vi "robot_object_test.vi"() -> ()   [LabVIEW 2009]
uses:
  OGRE/nick/FPGA/behaviors/driveable paths/test variable.vi
panel:
  in  "number 16\" iterations":i32
  in  "y LIDAR position":i16
  in  "x LIDAR position":i16
  out "Y positions":i16[](array[numeric])
  out "x positions":i16[](array[numeric])
  out "XY Graph":cluster{"Y":dbl[], "Y":dbl[]}[](graph)
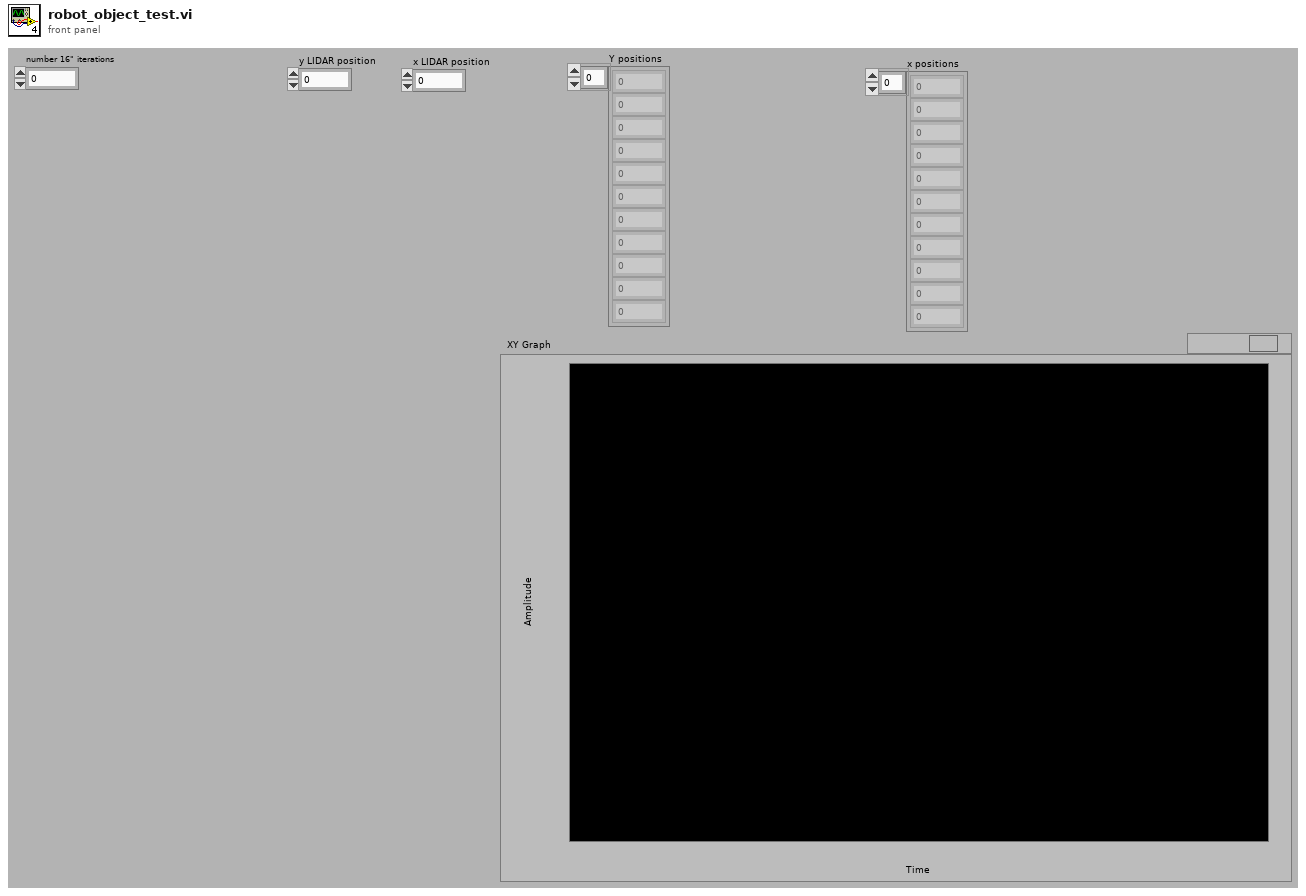
[diagram p1: front panel]
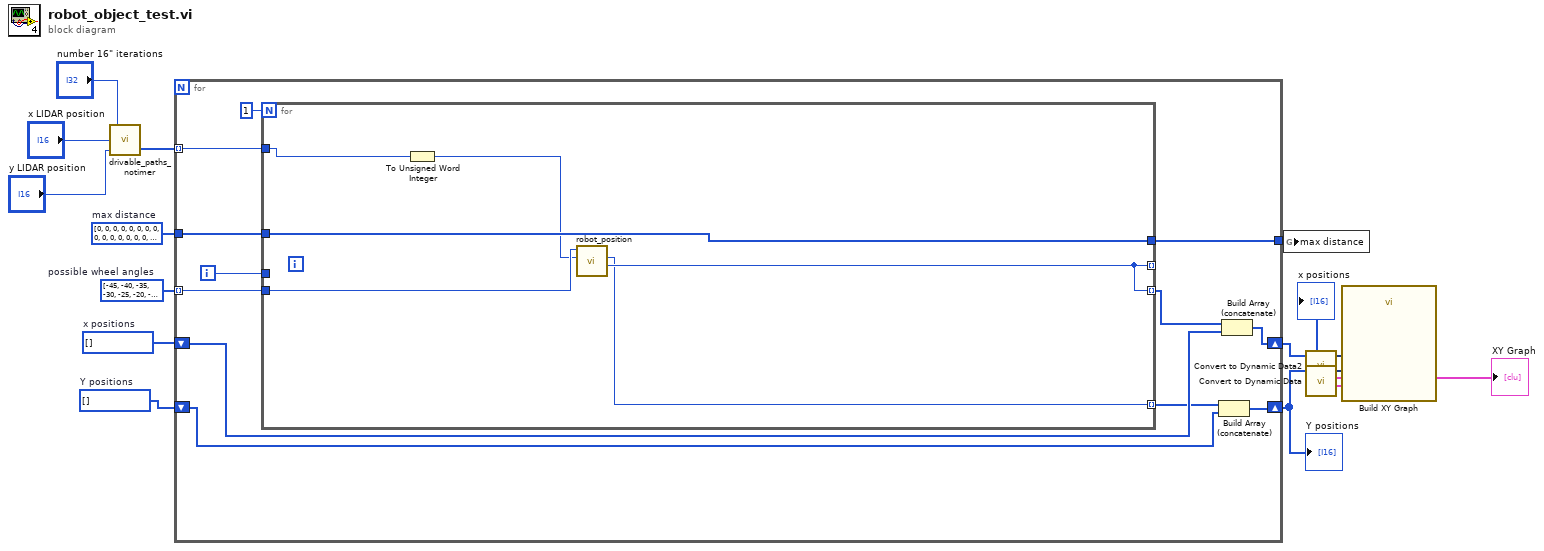
[diagram p0: block diagram]
diagram:
  w9 = i16[] []  # Y positions
  w10 = i16[] []  # x positions
  w12 = i8[] [-45, -40, -35, -30, -25, -20, -15, -10, -5, 0, 5, 10, 15, 20, 25, 30, 35, 40, 45]  # possible wheel angles
  w13 = i16[] [0, 0, 0, 0, 0, 0, 0, 0, 0, 0, 0, 0, 0, 0, 0, 0, 0, 0, 0]  # max distance
  n1 = call "drivable_paths_notimer.vi"("y LIDAR position"="y LIDAR position", "x LIDAR position"="x LIDAR position", "number 16\" iterations"="number 16\" iterations") -> ("max distance"=w4:i16[])  [unwired: 1 in]
  n2 = for {
    tunnel: w13 -> [w26]
    tunnel: w12 -> [w17] mode=indexing
    tunnel: [w24] -> w11
    shift-right: [w21] -> w6
    shift-left: w10 -> [w22]
    shift-right: [w20] -> w8
    shift-left: w9 -> [w18]
    tunnel: w4 -> [w16] mode=indexing
    i -> [w25]
    n3 = for {
      N: 1 -> [_]
      tunnel: w26 -> [w31]
      tunnel: [w31] -> w24
      tunnel: w25 -> [_]
      tunnel: w17 -> [w32]
      tunnel: [w30] -> _ mode=indexing
      tunnel: [w30] -> w23 mode=indexing
      tunnel: [w29] -> w19 mode=indexing
      tunnel: w16 -> [w28]
      n4 = To Unsigned Word Integer(number=w28) -> (unsigned 16bit integer=w27:u16)
      n5 = call "robot_position.vi"("Distance Along Arc"=w27, "Wheel Angle"=w32) -> ("New X Position"=w30:i8, "New Y Position"=w29:i8)  [unwired: 7 in, 1 out]
    }
    n6 = Build Array (concatenate)(w19, w18) -> (w20:i16[])
    n7 = Build Array (concatenate)(w23, w22) -> (w21:i16[])
  }
  "x positions" <- w6
  "Y positions" <- w8
  n8 = global write "test variable.vi" "max distance"(w11) -> ()
  n9 = call "Convert to Dynamic Data2"("Array"=w6) -> ("Dynamic Data Type"=w5:dynamicdata)  [unwired: 3 in]
  n10 = call "Convert to Dynamic Data"("Array"=w8) -> ("Dynamic Data Type"=w7:dynamicdata)  [unwired: 3 in]
  n11 = call "Build XY Graph"("Y Input"=w7, "X Input"=w5) -> ("XY Graph"=→"XY Graph":cluster{"Y":dbl[], "Y":dbl[]}[])  [unwired: 8 in, 1 out]
